vi "niSYS UTIL Create Exports -myPC.vi"() -> ()   [LabVIEW 2017]
doc: "This is the scripting VI that will create a set or get VI to compliment a SEQ class. It demonstrates the power of scripting. Additionally it could be further customized for a development team. For instance the user must select set/get before runnning the VI. This could be modified to simplify usage.\n\nAAL 9/09"
uses:
  <vilib>/Utility/traverseref.llb/TRef TravTarget.ctl
  <vilib>/Utility/miscctls.llb/LVPositionTypeDef.ctl
panel:
  in  "Cancel Button":bool
  in  "Object DataRef Path":path=path "C:/Users/mcsean/Desktop/cla/2012_AAL Exercises_ Solutions/ExerciseSource/By Reference Objects/SEQ Wind Turbine Object/Controls/Wind Turbine DataRef.ctl"
  out "error out":errorcluster
  in  "Create":bool
  in  "Set/Get (Set)":bool=TRUE
  in  "Object Data Elements":i32(listbox)
  # "Instructions:\n\n1. Select type of Export: Set or Get\n2. Select the Measurement Handle\n3. Run the VI.\n4. Select the State Element Item to create an export from\n5. Press Create Export to finish\n6. The Export will be open but not saved.\n7. If is a Get export, fix the tunnel value for false case.\n8. Save the Export"
  # "Set\n\nGet"
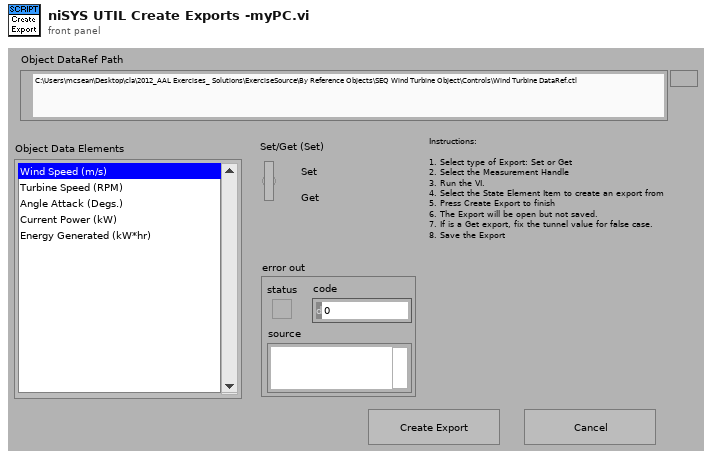
[diagram p1: front panel]
types:
  T1 = enum32{"Invalid", "Standard", "Closed", "Hidden", "Minimized", "Maximized"}
  T2 = typedef "TRef TravTarget.ctl" = enum16{"FP", "BD", "Other"}
  T3 = typedef "LVPositionTypeDef.ctl" = cluster{"Left":i32, "Top":i32}
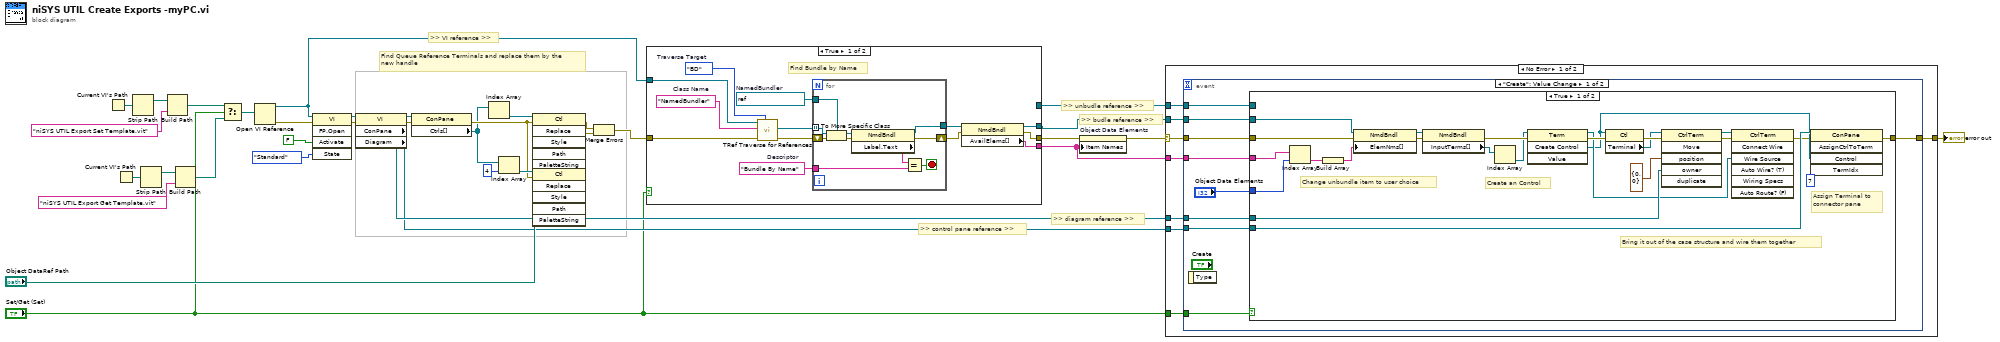
[diagram p0: block diagram]
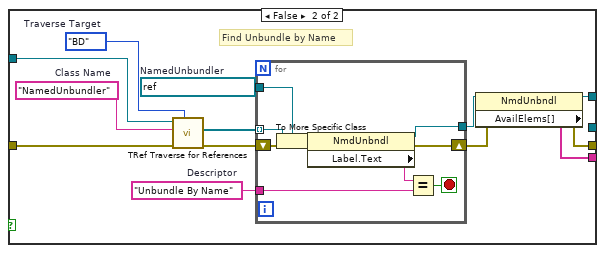
[diagram p2: hidden frame]
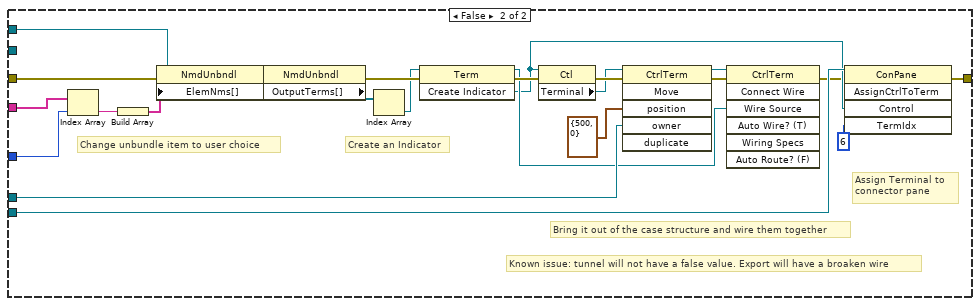
[diagram p3: hidden frame]
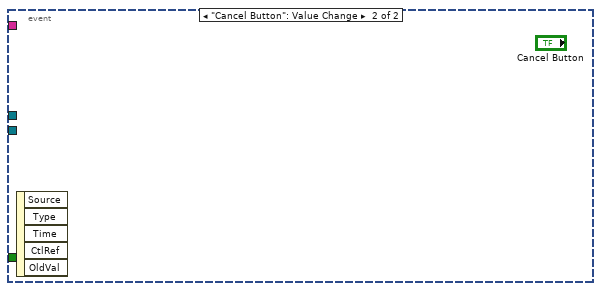
[diagram p4: hidden frame]
diagram:
  # ">> unbudle reference >>"
  # ">> budle reference >>"
  # ">> VI reference >>"
  # ">> diagram reference >>"
  # ">> control pane reference >>"
  # "Find Queue Reference Terminals and replace them by the\nnew handle"
  n1 = Current VI's Path() -> (path=w18:path)
  n2 = Current VI's Path() -> (path=w9:path)
  n3 = Strip Path(path=w18) -> (stripped path=w17:path)  [unwired: 1 out]
  n4 = Strip Path(path=w9) -> (stripped path=w10:path)  [unwired: 1 out]
  n5 = Build Path(base path=w17, name or relative path="niSYS UTIL Export Set Template.vit") -> (appended path=w15:path)
  n6 = Build Path(base path=w10, name or relative path="niSYS UTIL Export Get Template.vit") -> (appended path=w8:path)
  n7 = Select(t=w15, s="Set/Get (Set)", f=w8) -> (s? t:f=w34:path)
  n8 = Open VI Reference(vi path=w34) -> (vi reference=w6:refnum<vi>, error out=w33:errorcluster)  [unwired: 1 in, 4 out]
  n9 = invoke class="VI" method="FP.Open"(reference=w6, error in=w33, "Activate"=FALSE ("Activate?"), "State"=T1."Standard") -> (reference out=w13:refnum<vi>, error out=w30:errorcluster)  [unwired: 1 in, 3 out]
  n10 = property class="VI"(reference=w13, error in=w30) -> (error out=w29:errorcluster, "ConPane"=w12:refnum<vi>, "Diagram"=w20:refnum<vi>)  [unwired: 1 out]
  n11 = property class="ConPane"(reference=w12, error in=w29) -> (error out=w25:errorcluster, "Ctrls[]"=w11:refnum<vi>[])  [unwired: 1 out]
  n12 = Index Array(array=w11) -> (element=w28:refnum<vi>)  [unwired: 1 in]
  n13 = Index Array(array=w11, index=4) -> (element=w26:refnum<vi>)
  n14 = invoke class="Ctl" method="Replace"(reference=w28, error in=w25, "Path"="Object DataRef Path") -> (error out=w23:errorcluster)  [unwired: 3 in, 5 out]
  n15 = invoke class="Ctl" method="Replace"(reference=w26, error in=w25, "Path"="Object DataRef Path") -> (error out=w22:errorcluster)  [unwired: 3 in, 5 out]
  n16 = Merge Errors(w23, w22) -> (w21:errorcluster)
  n17 = case shown="True" "Set/Get (Set)" {
    tunnel: w21 -> [w47 w70]
    tunnel: [w36 w61] -> w4
    tunnel: [w37 _] -> w3
    tunnel: w6 -> [w40 w63]
    tunnel: [w35 w59] -> w5
    tunnel: [_ w58] -> w2
    frame True {
      w42 = refnum<vi> refnum  # NamedBundler
      w44 = "NamedBundler"  # Class Name
      w45 = TRef_TravTarget."BD"  # Traverse Target
      w46 = "Bundle By Name"  # Descriptor
      # "Find Bundle by Name"
      n18 = call <vilib>:"TRef Traverse for References.vi"("Traverse Target"=w45, "error in (no error)"=w47, "Class Name"=w44, "VI Refnum"=w40) -> ("error out"=w41:errorcluster, "References"=w43:refnum<vi>[])  [unwired: 1 in, 5 out]
      n19 = for {
        tunnel: w43 -> [w57] mode=indexing
        tunnel: w42 -> [w56]
        tunnel: [w54] -> w39
        shift-right: [w53] -> w38
        shift-left: w41 -> [w52]
        tunnel: w46 -> [w50]
        stop <- w48 stop-if-true
        n20 = To More Specific Class(target class=w56, reference=w57, error in=w52) -> (specific class reference=w55:refnum<vi>, error out=w51:errorcluster)
        n21 = property class="NmdBndl"(reference=w55, error in=w51) -> (reference out=w54:refnum<vi>, error out=w53:errorcluster, "Label.Text"=w49:string)
        n22 = Equal?(x=w49, y=w50) -> (x = y?=w48:bool)
      }
      n23 = property class="NmdBndl"(reference=w39, error in=w38) -> (reference out=w37:refnum<vi>, error out=w36:errorcluster, "AvailElems[]"=w35:string[])
    }
    frame False {
      w65 = refnum<vi> refnum  # NamedUnbundler
      w67 = "NamedUnbundler"  # Class Name
      w68 = TRef_TravTarget."BD"  # Traverse Target
      w69 = "Unbundle By Name"  # Descriptor
      # "Find Unbundle by Name"
      n24 = call <vilib>:"TRef Traverse for References.vi"("Traverse Target"=w68, "error in (no error)"=w70, "Class Name"=w67, "VI Refnum"=w63) -> ("error out"=w64:errorcluster, "References"=w66:refnum<vi>[])  [unwired: 1 in, 5 out]
      n25 = for {
        tunnel: w66 -> [w80] mode=indexing
        tunnel: w65 -> [w79]
        tunnel: [w77] -> w60
        shift-right: [w76] -> w62
        shift-left: w64 -> [w75]
        tunnel: w69 -> [w73]
        stop <- w71 stop-if-true
        n26 = To More Specific Class(target class=w79, reference=w80, error in=w75) -> (specific class reference=w78:refnum<vi>, error out=w74:errorcluster)
        n27 = property class="NmdUnbndl"(reference=w78, error in=w74) -> (reference out=w77:refnum<vi>, error out=w76:errorcluster, "Label.Text"=w72:string)
        n28 = Equal?(x=w72, y=w73) -> (x = y?=w71:bool)
      }
      n29 = property class="NmdUnbndl"(reference=w60, error in=w62) -> (reference out=w58:refnum<vi>, error out=w61:errorcluster, "AvailElems[]"=w59:string[])
    }
  }
  n30 = property on="Object Data Elements" class="LstBox (strict)"(error in=w4, "Item Names"=w5) -> (error out=w14:errorcluster)  [unwired: 1 in, 1 out]
  n31 = case shown="No Error" w14 {
    selector: w14 -> [w84 w146]
    tunnel: w5 -> [w88 _]
    tunnel: w3 -> [w87 _]
    tunnel: w20 -> [w86 _]
    tunnel: [w85 w146] -> w19
    tunnel: w12 -> [w83 _]
    tunnel: w2 -> [w82 _]
    tunnel: "Set/Get (Set)" -> [w81 _]
    frame No Error {
      n32 = event shown="[0] \"Create\": Value Change" {
        selector: _ -> [_ _]
        dyn-events: _ -> [_ _]
        timeout: _ -> [_ _]
        tunnel: w88 -> [w97 _]
        tunnel: w87 -> [w96 _]
        tunnel: w84 -> [w95 _]
        tunnel: w86 -> [w94 _]
        tunnel: [w92 _] -> w85
        tunnel: w83 -> [w93 _]
        tunnel: w82 -> [w89 _]
        tunnel: w81 -> [w91 _]
        event "Create": Value Change {
          n33 = event-data() -> ()  [unwired: 2 out]
          n34 = case shown="True" w91 {
            tunnel: w97 -> [w121 w145]
            tunnel: w96 -> [w120 _]
            tunnel: w95 -> [w117 w142]
            tunnel: w94 -> [w110 w135]
            tunnel: w93 -> [w103 w128]
            tunnel: [w100 w125] -> w92
            tunnel: "Object Data Elements" -> [w98 w123]
            tunnel: w89 -> [_ w122]
            frame True {
              # "Assign Terminal to \nconnector pane"
              # "Bring it out of the case structure and wire them together"
              # "Create an Control"
              # "Change unbundle item to user choice"
              n35 = Index Array(array=w121, index=w98) -> (element=w119:string)
              n36 = Build Array(w119) -> (w118:string[])
              n37 = property class="NmdBndl"(reference=w120, error in=w117, "ElemNms[]"=w118) -> (reference out=w114:refnum<vi>, error out=w116:errorcluster)
              n38 = property class="NmdBndl"(reference=w114, error in=w116) -> (error out=w113:errorcluster, "InputTerms[]"=w115:refnum<vi>[])  [unwired: 1 out]
              n39 = Index Array(array=w115) -> (element=w107:refnum<vi>)  [unwired: 1 in]
              n40 = invoke class="Term" method="Create Control"(reference=w107, error in=w113) -> (reference out=w105:refnum<vi>, error out=w111:errorcluster, "Create Control"=w102:refnum<vi>)  [unwired: 2 in, 1 out]
              n41 = property class="Ctl"(reference=w102, error in=w111) -> (error out=w112:errorcluster, "Terminal"=w109:refnum<vi>)  [unwired: 1 out]
              n42 = invoke class="CtrlTerm" method="Move"(reference=w109, error in=w112, "position"=T3 {"Left"=0, "Top"=0}, "owner"=w110) -> (reference out=w106:refnum<vi>, error out=w104:errorcluster)  [unwired: 2 in, 4 out]
              n43 = invoke class="CtrlTerm" method="Connect Wire"(reference=w106, error in=w104, "Wire Source"=w105) -> (error out=w101:errorcluster)  [unwired: 4 in, 6 out]
              n44 = invoke class="ConPane" method="AssignCtrlToTerm"(reference=w103, error in=w101, "Control"=w102, "TermIdx"=u32 7 ("Terminal Index")) -> (error out=w100:errorcluster)  [unwired: 1 in, 4 out]
            }
            frame False {
              # "Assign Terminal to \nconnector pane"
              # "Known issue: tunnel will not have a false value. Export will have a broaken wire"
              # "Bring it out of the case structure and wire them together"
              # "Create an Indicator"
              # "Change unbundle item to user choice"
              n45 = Index Array(array=w145, index=w123) -> (element=w144:string)
              n46 = Build Array(w144) -> (w143:string[])
              n47 = property class="NmdUnbndl"(reference=w122, error in=w142, "ElemNms[]"=w143) -> (reference out=w139:refnum<vi>, error out=w141:errorcluster)
              n48 = property class="NmdUnbndl"(reference=w139, error in=w141) -> (error out=w138:errorcluster, "OutputTerms[]"=w140:refnum<vi>[])  [unwired: 1 out]
              n49 = Index Array(array=w140) -> (element=w132:refnum<vi>)  [unwired: 1 in]
              n50 = invoke class="Term" method="Create Indicator"(reference=w132, error in=w138) -> (reference out=w130:refnum<vi>, error out=w136:errorcluster, "Create Indicator"=w127:refnum<vi>)  [unwired: 1 in]
              n51 = property class="Ctl"(reference=w127, error in=w136) -> (error out=w137:errorcluster, "Terminal"=w134:refnum<vi>)  [unwired: 1 out]
              n52 = invoke class="CtrlTerm" method="Move"(reference=w134, error in=w137, "position"=T3 {"Left"=500, "Top"=0}, "owner"=w135) -> (reference out=w131:refnum<vi>, error out=w129:errorcluster)  [unwired: 2 in, 4 out]
              n53 = invoke class="CtrlTerm" method="Connect Wire"(reference=w131, error in=w129, "Wire Source"=w130) -> (error out=w126:errorcluster)  [unwired: 4 in, 6 out]
              n54 = invoke class="ConPane" method="AssignCtrlToTerm"(reference=w128, error in=w126, "Control"=w127, "TermIdx"=u32 6 ("Terminal Index")) -> (error out=w125:errorcluster)  [unwired: 1 in, 4 out]
            }
          }
        }
        event "Cancel Button": Value Change {
          n55 = event-data() -> ()  [unwired: 6 out]
        }
      }
    }
    frame Error {
    }
  }
  "error out" <- w19
